vi "DSF.Shared.Configuration.Execution Timing.Is Active.vi"(8 "error in (no error)":errorcluster, 10 "iteration":u64=1, 11 "Execution Timing in":refnum<class "DSF.Engine.Timing.lvclass">) -> (0 "error out":errorcluster, 2 "active?":bool, 3 "Execution Timing out":refnum<class "DSF.Engine.Timing.lvclass">)   [LabVIEW 2016, in "DSF.Engine.lvlib" / "DSF.Engine.Timing.lvclass"]
uses:
  DSF.Engine.Timing.lvclass
  DSF.Engine.Timing.lvclass/DSF.Engine.Timing.ctl
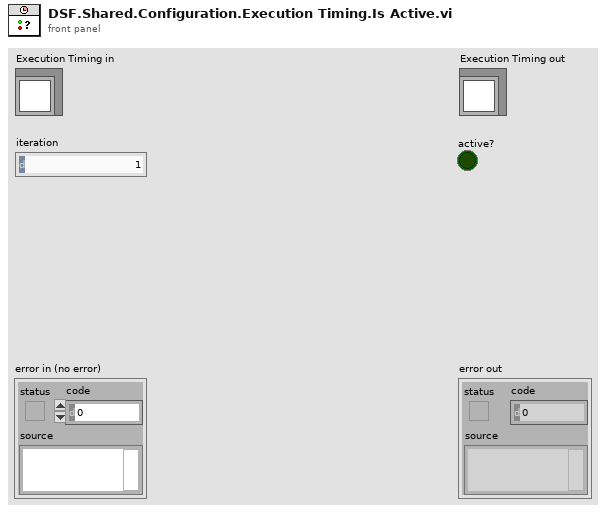
[diagram p1: front panel]
types:
  T1 = typedef "DSF.Shared.lvlib/DSF.Shared.Typedefs.Scalars.Decimation.ctl" = u64
  T2 = typedef "DSF.Shared.lvlib/DSF.Shared.Typedefs.Scalars.Offset.ctl" = u64
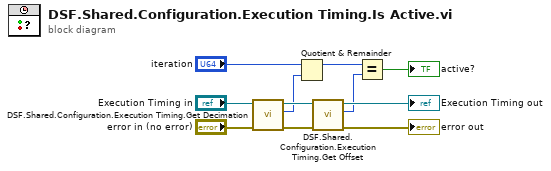
[diagram p0: block diagram]
diagram:
  n1 = call "DSF.Shared.Configuration.Execution Timing.Get Decimation.vi"("error in (no error)"="error in (no error)", "DSF.Shared.Configuration.Execution Timing in"="Execution Timing in") -> ("error out"=w8:errorcluster, "Decimation"=w4:T1, "DSF.Shared.Configuration.Execution Timing out"=w9:refnum<class "DSF.Engine.Timing.lvclass">)  [unwired: 7 in]
  n2 = Quotient & Remainder(x="iteration", y=w4) -> (x-y*floor(x/y)=w7:T1)  [unwired: 1 out]
  n3 = call "DSF.Shared.Configuration.Execution Timing.Get Offset.vi"("error in (no error)"=w8, "DSF.Shared.Configuration.Execution Timing in"=w9) -> ("error out"=→"error out":errorcluster, "Offset"=w5:T2, "DSF.Shared.Configuration.Execution Timing out"=→"Execution Timing out":refnum<class "DSF.Engine.Timing.lvclass">)  [unwired: 7 in]
  n4 = Equal?(x=w7, y=w5) -> (x = y?=→"active?":bool)
